vi "PMW_ TCRT5000.vi"() -> ()   [LabVIEW 2020]
uses:
  <vilib>/MakerHub/LINX/Public/Peripherals/Digital/Digital Read 1 Chan.vi
  <vilib>/MakerHub/LINX/Public/Peripherals/Digital/Digital Read N Chans.vi
  <vilib>/MakerHub/LINX/Private/Local IO/LinxDigitalRead.vi
  <vilib>/MakerHub/LINX/Public/Utilities/Check Channel.vi
  <vilib>/MakerHub/LINX/Public/Utilities/Open Serial.vi
  <vilib>/MakerHub/LINX/Private/Utilties/Generate Error.vi
  <vilib>/MakerHub/LINX/LMH-LINX.lvlib
  <vilib>/ptbypt/NI_PtbyPt.lvlib
panel:
  out "Contador de Pulsos":dbl
  out "RPM":dbl
  out "Pulsos por minuto":dbl
  in  "?":bool
  in  "Digital Channel":u8
  in  "Serial Port":refnum<visa-resource-name>
  in  "Pulsos*Rev":dbl
  out "Revoluciones por minuto":dbl(knob) scale=0.0..100.0
  out "Pulso":bool
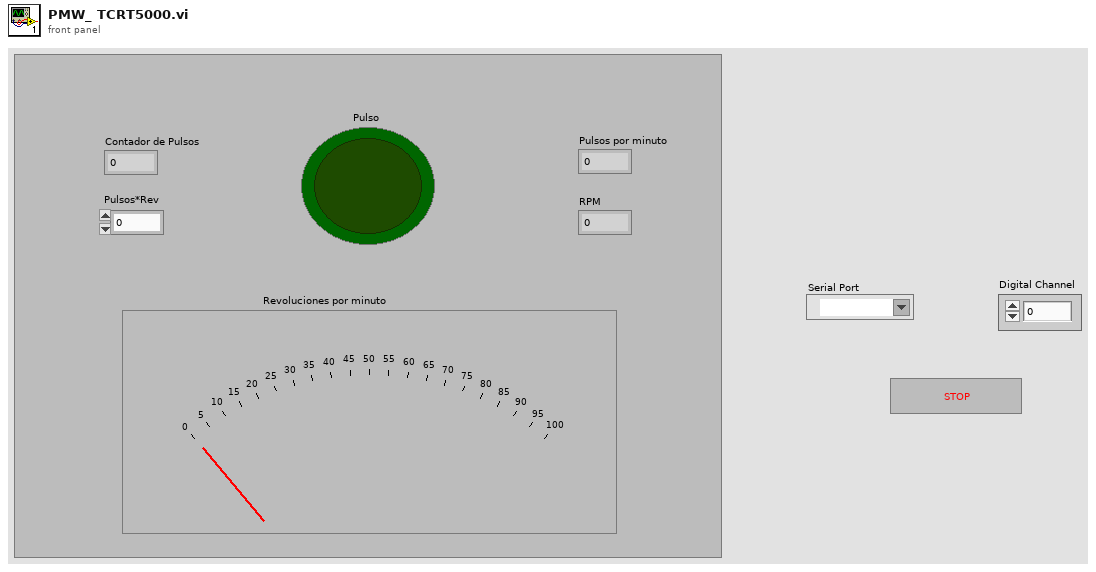
[diagram p1: front panel]
types:
  T1 = typedef "LMH-LINX.lvlib/LINX Ref.ctl" = cluster{"IO":T2, "Interface":T3, "LINX Device Config":T4}
  T2 = typedef "LMH-LINX.lvlib/Platform.ctl" = enum16{"Remote", "Local"}
  T3 = typedef "LMH-LINX.lvlib/Interface.ctl" = enum16{"Serial", "TCP"}
  T4 = typedef "LMH-LINX.lvlib/Device.lvlib/LINX Device Config.ctl" = cluster{"Interface":T3, "COM Port":refnum<visa-resource-name>, "TCP Configuration":T5, "Device Family":u8, "Device ID":u8, "Device Name":string, "TCP Ref":refnum<k5>, "Channels":T6}
  T5 = typedef "LMH-LINX.lvlib/Device.lvlib/TCP Config.ctl" = cluster{"IP Address":string, "Port":u16}
  T6 = typedef "LMH-LINX.lvlib/Channels.ctl" = cluster{"DI":u8[], "DO":u8[], "AI":u8[], "AO":u8[], "PWM":u8[], "QE":u8[], "UART":u8[], "I2C 2":u8[], "SPI":u8[], "CAN":u8[], "Servo":u8[], "AI Ref (V)":dbl, "AI Resolution (Bits)":u8, "AO Ref (V)":dbl, "AO Resolution (Bits)":u8}
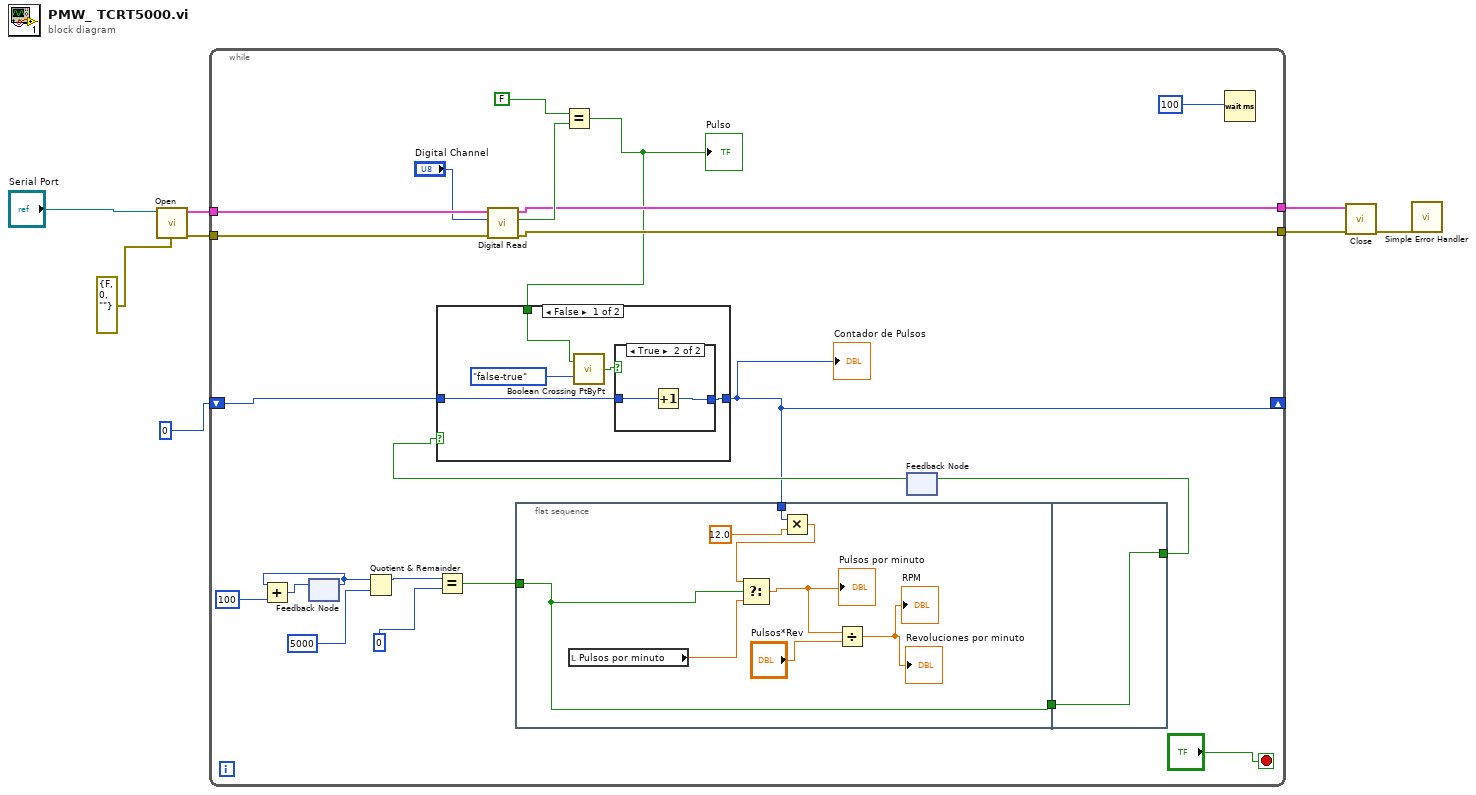
[diagram p0: block diagram]
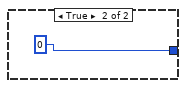
[diagram p3: hidden frame]
diagram:
  n1 = call-poly <vilib>:"Open.vi"("Error In"=errorcluster {"status"=FALSE, "code"=0, "source"=""} ("error constant"), "Serial Port"="Serial Port") -> ("Error Out"=w5:errorcluster, "LINX Resource"=w6:T1)  [unwired: 7 in, 1 out]
  n2 = while {
    tunnel: w6 -> [w29]
    tunnel: w5 -> [w28]
    tunnel: [w19] -> w3
    tunnel: [w18] -> w2
    shift-right: [w11] -> _
    shift-left: 0 -> [w12]
    stop <- "?" stop-if-true
    n3 = feedback #1() -> (w22:i32)  [unwired: 1 in]
    n4 = Add(x=w22, y=100) -> (x+y=w23:i32)
    n5 = feedback-in #1(w23) -> ()
    n6 = Quotient & Remainder(x=w22, y=5000) -> (x-y*floor(x/y)=w9:i32)  [unwired: 1 out]
    n7 = Equal?(x=w9, y=0) -> (x = y?=w10:bool)
    n8 = call-poly <vilib>:"Digital Read.vi"("Error In"=w28, "DI Channel"="Digital Channel", "LINX Resource"=w29) -> ("Error Out"=w18:errorcluster, "DI Value"=w25:bool, "LINX Resource"=w19:T1)  [unwired: 6 in]
    n9 = flat-sequence {
      tunnel: w11 -> [w33]
      tunnel: [w31] -> w16
      tunnel: w10 -> [w31]
      tunnel: w16 -> [w39]
      tunnel: [w39] -> w15
      frame #0 {
        n10 = local read "Pulsos por minuto"() -> (w32:dbl)
        n11 = Multiply(x=w33, y=12.0) -> (x*y=w38:dbl)
        n12 = Select(t=w38, s=w31, f=w32) -> (s? t:f=w36:dbl)
        "Pulsos por minuto" <- w36
        n13 = Divide(x=w36, y="Pulsos*Rev") -> (x/y=→"RPM" →"Revoluciones por minuto":dbl)
      }
      frame #1 {
      }
    }
    n14 = Equal?(x=FALSE, y=w25) -> (x = y?=w13:bool)
    "Pulso" <- w13
    n15 = feedback-in #2(w15) -> ()
    n16 = feedback #2() -> (w14:bool)  [unwired: 1 in]
    n17 = case shown="False" w14 {
      tunnel: [w44 0] -> w11
      tunnel: w12 -> [w43 _]
      tunnel: w13 -> [w41 _]
      frame False {
        n18 = call <vilib>:"Boolean Crossing PtByPt.vi"("direction"=enum16{"either", "false-true", "true-false"}."false-true", "input"=w41) -> ("crossing"=w42:bool)  [unwired: 1 in]
        n19 = case shown="True" w42 {
          tunnel: [w45 w47] -> w44
          tunnel: w43 -> [w45 w46]
          frame False {
          }
          frame True {
            n20 = Increment(x=w46) -> (x+1=w47:i32)
          }
        }
      }
      frame True {
      }
    }
    "Contador de Pulsos" <- w11
    n21 = Wait (ms)(milliseconds to wait=100) -> ()  [unwired: 1 out]
  }
  n22 = call <vilib>:"Close.vi"("Error In"=w2, "LINX Resource"=w3) -> ("Error Out"=w4:errorcluster)  [unwired: 9 in]
  n23 = call <vilib>:"Simple Error Handler.vi"("error in (no error)"=w4) -> ()  [unwired: 4 in, 5 out]
